vi "Add Response.vi"   [LabVIEW 2019, in "Scripting API.lvlib"]
uses:
  Scripting API.lvlib
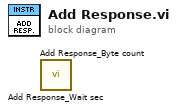
[diagram p0: block diagram]
diagram:
  n1 = call "Add Response_Wait sec.vi"() -> ()  [unwired: 9 in, 3 out]
  n2 = call "Add Response_Byte count.vi"() -> ()  [unwired: 9 in, 3 out]
